vi "Get_Channels_Map.vi"(3 "error in":errorcluster, 5 "Filename (.ini)":string="channels_map_default.ini") -> (0 "error out":errorcluster, 2 "Channels Map":T1)   [LabVIEW 2021]
uses:
  Channels_Map.ctl
  Channel_Cluster.ctl
  <vilib>/Utility/config.llb/Read Key (U32).vi
  <vilib>/Utility/config.llb/NI_LVConfig.lvlib
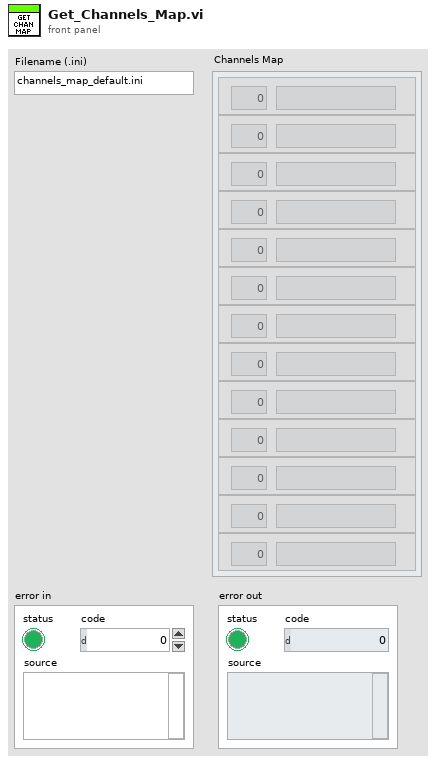
[diagram p1: front panel]
types:
  T1 = typedef "Channels_Map.ctl" = T2[]
  T2 = typedef "Channel_Cluster.ctl" = cluster{"Channel name":string, "Channel":u8}
  T3 = typedef "NI_LVConfig.lvlib/Config Data RefNum.ctl" = refnum<k1>
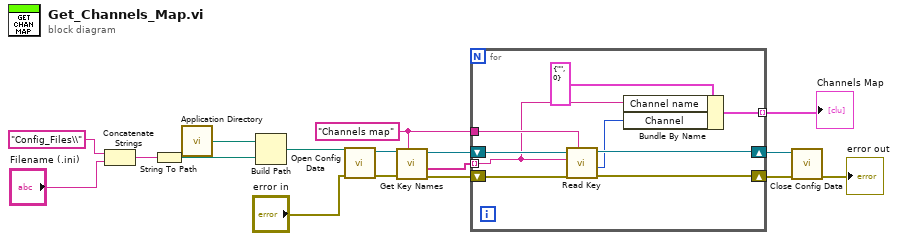
[diagram p0: block diagram]
diagram:
  w12 = "Channels map" ("section")
  n1 = Concatenate Strings("Config_Files\\" ("string"), "Filename (.ini)") -> (w4:string)
  n2 = String To Path(string=w4) -> (path=w6:path)
  n3 = call <vilib>:"Application Directory.vi"() -> ("Application Directory"=w7:path)
  n4 = Build Path(base path=w7, name or relative path=w6) -> (appended path=w3:path)
  n5 = call <vilib>:"Open Config Data.vi"("error in (no error)"="error in", "configuration file path"=w3) -> ("error out"=w16:errorcluster, "refnum"=w17:T3)  [unwired: 7 in, 1 out]
  n6 = call <vilib>:"Get Key Names.vi"("section"=w12, "error in (no error)"=w16, "refnum"=w17) -> ("error out"=w14:errorcluster, "key names"=w13:string[], "refnum out"=w15:T3)  [unwired: 5 in, 1 out]
  n7 = for {
    shift-right: [w23] -> w9
    shift-left: w15 -> [w24]
    shift-right: [w25] -> w10
    shift-left: w14 -> [w26]
    tunnel: w13 -> [w20] mode=indexing
    tunnel: w12 -> [w22]
    tunnel: [w18] -> w11 mode=indexing
    n8 = call-poly <vilib>:"Read Key.vi"("section"=w22, "error in (no error)"=w26, "key"=w20, "refnum"=w24) -> ("error out"=w25:errorcluster, "value"=w19:u32, "refnum out"=w23:T3)  [unwired: 4 in, 1 out]
    n9 = Bundle By Name(cluster=T2 {"Channel name"="", "Channel"=0} ("Channel Cluster"), "Channel name"=w20, "Channel"=w19) -> (w18:T2)
  }
  "Channels Map" <- w11
  n10 = call <vilib>:"Close Config Data.vi"("error in (no error)"=w10, "refnum"=w9) -> ("error out"=→"error out":errorcluster)  [unwired: 8 in, 1 out]
